vi "getCamSession.vi"(8 "error in":errorcluster, 10 "Camera name":T3, 11 "Input cluster":T1) -> (0 "error out":errorcluster, 1 "Width":u32, 2 "Height":u32, 3 "Output cluster":T1)   [LabVIEW 2020]
doc: "Create cam session for given Camera"
uses:
  <vilib>/userDefined/High Color/IMAQdx.ctl
  controls/StateMachineVariables.ctl
  <vilib>/vision/Avi.llb/IMAQ AVI2 Refnum.ctl
  <vilib>/vision/Deep Learning.llb/IMAQ DL Model Refnum.ctl
  <vilib>/vision/Image Controls.llb/IMAQ Image.ctl
  <vilib>/vision/driver/NI_Vision_Acquisition_Software.lvlib
  <resource>/objmgr/imaqdx.rc
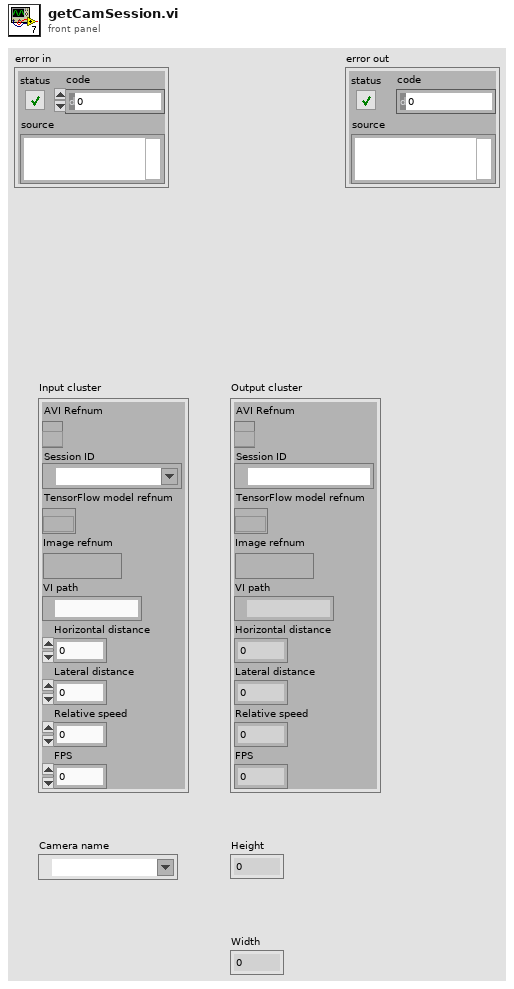
[diagram p1: front panel]
types:
  T1 = typedef "StateMachineVariables.ctl" = cluster{"AVI Refnum":T2, "Session ID":T3, "TensorFlow model refnum":T4, "Image refnum":T5, "VI path":path, "Horizontal distance":dbl, "Lateral distance":dbl, "Relative speed":dbl, "FPS":dbl}
  T2 = typedef "IMAQ AVI2 Refnum.ctl" = refnum<k20>
  T3 = typedef "IMAQdx.ctl" = refnum<k21>
  T4 = typedef "IMAQ DL Model Refnum.ctl" = refnum<k20>
  T5 = typedef "IMAQ Image.ctl" = refnum<image>
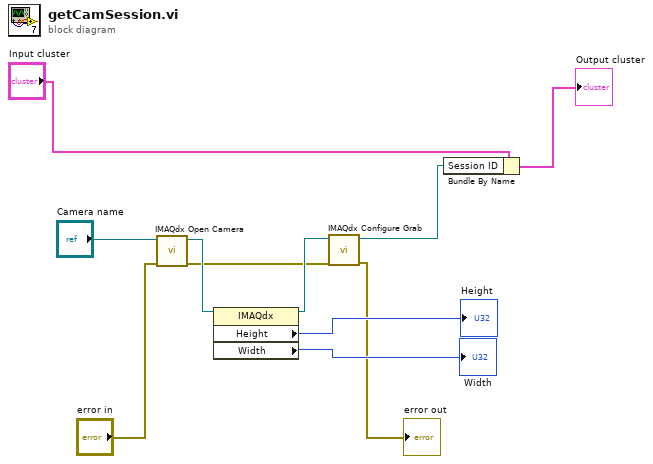
[diagram p0: block diagram]
diagram:
  n1 = call <vilib>:"IMAQdx Open Camera.vi"("error in"="error in", "Session In"="Camera name") -> ("error out"=w3:errorcluster, "Session Out"=w8:T3)  [unwired: 1 in, 7 out]
  n2 = property class="IMAQdx"(reference=w8) -> (reference out=w7:T3, "Height"=→"Height":u32, "Width"=→"Width":u32)  [unwired: 1 in, 1 out]
  n3 = call <vilib>:"IMAQdx Configure Grab.vi"("error in"=w3, "Session In"=w7) -> ("error out"=→"error out":errorcluster, "Session Out"=w4:T3)  [unwired: 8 in]
  n4 = Bundle By Name(cluster="Input cluster", "Session ID"=w4) -> (→"Output cluster":T1)
